vi "After Launch Init Core.vi"(8 "error in (no error)":errorcluster, 11 "BNT_DAQmx-MCSV-DOPWM in":refnum<class "BNT_DAQmx-MCSV-DOPWM.lvclass">) -> (0 "error out":errorcluster, 3 "BNT_DAQmx-MCSV-DOPWM out":refnum<class "BNT_DAQmx-MCSV-DOPWM.lvclass">)   [LabVIEW 2017, in "BNT_DAQmx.lvlib" / "BNT_DAQmx-MCSV-DOPWM.lvclass"]
doc: "Use <b>Pre Launch init.vi</b> method for sanity checks that are supposed to prevent the actor from launching if they fail. Use <B>this</B> method instead to initialize this actor when it has been activated. A corresponding high priority message will become dispatched before the <B>Actor Core.vi</b> is called.\n\n<b>Derived classed should call the parent methode first</b> and their own initialization code after.\n\nRefer also to the ongoing discussion at https://decibel.ni.com/content/message/57394#57394."
uses:
  BNT_DAQmx-MCSV-DOPWM.lvclass
  BNT_DAQmx-MCSV-DOPWM.lvclass/BNT_DAQmx-MCSV-DOPWM.ctl
  BNT_DAQmx-MCSV/BNT_DAQmx-MCSV.lvclass
  CSPP_Core/Classes/CSPP_ProcessVariables/CSPP_ProcessVariables.lvlib
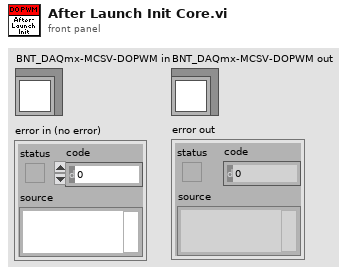
[diagram p1: front panel]
types:
  T1 = cluster{"Read Access":enum8{"Allowed", "Required", "None"}, "Write Access":enum8{"Allowed", "Required", "None"}}
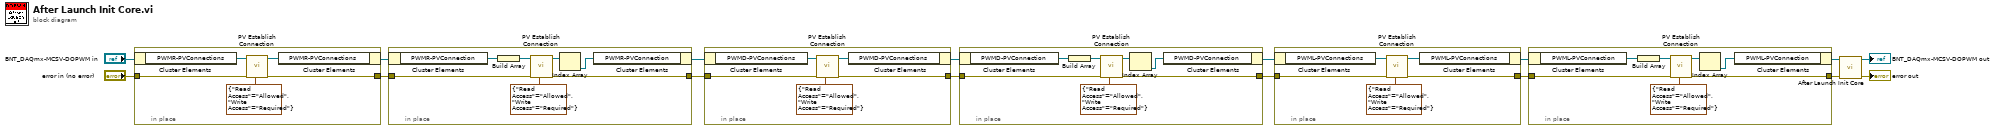
[diagram p0: block diagram]
diagram:
  n1 = in-place {
    in-place-border: [w18] -> w12
    in-place-border: "error in (no error)" -> [w21]
    n2 = in-place-cluster #1("BNT_DAQmx-MCSV-DOPWM in") -> ("PWMR-PVConnections"=w20:refnum<class "PVConnection.lvclass">[])
    n3 = call "PV Establish Connection.vi"("Access (R/W allowed)"=T1 {"Read Access"=enum."Allowed", "Write Access"=enum."Required"}, "Error In"=w21, "PVConnections in"=w20) -> ("Error Out"=w18:errorcluster, "PVConnections out"=w19:refnum<class "PVConnection.lvclass">[])  [unwired: 7 in]
    n4 = in-place-cluster #1("PWMR-PVConnections"=w19) -> (w11:refnum<class "BNT_DAQmx-MCSV-DOPWM.lvclass">)
  }
  n5 = in-place {
    in-place-border: [w25] -> w7
    in-place-border: w12 -> [w28]
    n6 = in-place-cluster #2(w11) -> ("PWMR-PVConnection"=w27:refnum<class "PVConnection.lvclass">)
    n7 = Build Array(w27) -> (w23:refnum<class "PVConnection.lvclass">[])
    n8 = call "PV Establish Connection.vi"("Access (R/W allowed)"=T1 {"Read Access"=enum."Allowed", "Write Access"=enum."Required"}, "Error In"=w28, "PVConnections in"=w23) -> ("Error Out"=w25:errorcluster, "PVConnections out"=w26:refnum<class "PVConnection.lvclass">[])  [unwired: 7 in]
    n9 = Index Array(array=w26) -> (element=w22:refnum<class "PVConnection.lvclass">)  [unwired: 1 in]
    n10 = in-place-cluster #2("PWMR-PVConnection"=w22) -> (w8:refnum<class "BNT_DAQmx-MCSV-DOPWM.lvclass">)
  }
  n11 = in-place {
    in-place-border: [w30] -> w9
    in-place-border: w7 -> [w33]
    n12 = in-place-cluster #3(w8) -> ("PWMD-PVConnections"=w32:refnum<class "PVConnection.lvclass">[])
    n13 = call "PV Establish Connection.vi"("Access (R/W allowed)"=T1 {"Read Access"=enum."Allowed", "Write Access"=enum."Required"}, "Error In"=w33, "PVConnections in"=w32) -> ("Error Out"=w30:errorcluster, "PVConnections out"=w31:refnum<class "PVConnection.lvclass">[])  [unwired: 7 in]
    n14 = in-place-cluster #3("PWMD-PVConnections"=w31) -> (w10:refnum<class "BNT_DAQmx-MCSV-DOPWM.lvclass">)
  }
  n15 = in-place {
    in-place-border: [w37] -> w4
    in-place-border: w9 -> [w40]
    n16 = in-place-cluster #4(w10) -> ("PWMD-PVConnection"=w39:refnum<class "PVConnection.lvclass">)
    n17 = Build Array(w39) -> (w35:refnum<class "PVConnection.lvclass">[])
    n18 = call "PV Establish Connection.vi"("Access (R/W allowed)"=T1 {"Read Access"=enum."Allowed", "Write Access"=enum."Required"}, "Error In"=w40, "PVConnections in"=w35) -> ("Error Out"=w37:errorcluster, "PVConnections out"=w38:refnum<class "PVConnection.lvclass">[])  [unwired: 7 in]
    n19 = Index Array(array=w38) -> (element=w34:refnum<class "PVConnection.lvclass">)  [unwired: 1 in]
    n20 = in-place-cluster #4("PWMD-PVConnection"=w34) -> (w3:refnum<class "BNT_DAQmx-MCSV-DOPWM.lvclass">)
  }
  n21 = in-place {
    in-place-border: [w42] -> w6
    in-place-border: w4 -> [w45]
    n22 = in-place-cluster #5(w3) -> ("PWML-PVConnections"=w44:refnum<class "PVConnection.lvclass">[])
    n23 = call "PV Establish Connection.vi"("Access (R/W allowed)"=T1 {"Read Access"=enum."Allowed", "Write Access"=enum."Required"}, "Error In"=w45, "PVConnections in"=w44) -> ("Error Out"=w42:errorcluster, "PVConnections out"=w43:refnum<class "PVConnection.lvclass">[])  [unwired: 7 in]
    n24 = in-place-cluster #5("PWML-PVConnections"=w43) -> (w5:refnum<class "BNT_DAQmx-MCSV-DOPWM.lvclass">)
  }
  n25 = in-place {
    in-place-border: [w49] -> w1
    in-place-border: w6 -> [w52]
    n26 = in-place-cluster #6(w5) -> ("PWML-PVConnection"=w51:refnum<class "PVConnection.lvclass">)
    n27 = Build Array(w51) -> (w47:refnum<class "PVConnection.lvclass">[])
    n28 = call "PV Establish Connection.vi"("Access (R/W allowed)"=T1 {"Read Access"=enum."Allowed", "Write Access"=enum."Required"}, "Error In"=w52, "PVConnections in"=w47) -> ("Error Out"=w49:errorcluster, "PVConnections out"=w50:refnum<class "PVConnection.lvclass">[])  [unwired: 7 in]
    n29 = Index Array(array=w50) -> (element=w46:refnum<class "PVConnection.lvclass">)  [unwired: 1 in]
    n30 = in-place-cluster #6("PWML-PVConnection"=w46) -> (w2:refnum<class "BNT_DAQmx-MCSV-DOPWM.lvclass">)
  }
  n31 = call-parent "After Launch Init Core.vi"("error in (no error)"=w1, "BNT_DAQmx-MCSV in"=w2) -> ("error out"=→"error out":errorcluster, "BNT_DAQmx-MCSV out"=→"BNT_DAQmx-MCSV-DOPWM out":refnum<class "BNT_DAQmx-MCSV-DOPWM.lvclass">)  [unwired: 8 in]
